vi "Begin.vi"(8 "error in (no error)":errorcluster, 10 "Config In":variant, 11 "TalonSRX in":refnum<class "TalonSRX.lvclass">) -> (0 "error out":errorcluster, 3 "TalonSRX out":refnum<class "TalonSRX.lvclass">)   [LabVIEW 2019, in "Drive.lvlib" / "TalonSRX.lvclass"]
uses:
  TalonSRX.lvclass
  C:/Users/Public/Documents/2020InfiniteRecharge/src robot/Classes/Drive/Tank Drive/Tank Drive.lvclass
  CTRE Drive.lvclass
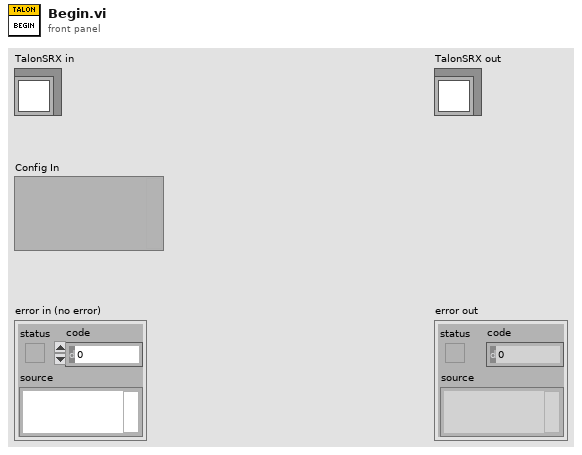
[diagram p1: front panel]
types:
  T1 = typedef "Drive.lvlib/Tank Drive.lvclass/Motor Controller IDs.ctl" = cluster{"Left Lead":u8, "Right Lead":u8, "Left Followers":u8[], "Right Followers":u8[]}
  T2 = typedef "Drive.lvlib/Tank Drive.lvclass/Motor Controller Names.ctl" = cluster{"Left Lead":string, "Right Lead":string, "Left Followers":string[], "Right Followers":string[]}
  T3 = typedef "CTRE_Phoenix_MotorControl_SlotStructure.ctl" = cluster{"P":dbl, "I":dbl, "D":dbl, "F":dbl, "integralZone":dbl, "allowableClosedLoopError":i32, "maxIntegralAccumulator":dbl, "closedLoopPeakOutput":dbl, "closedLoopPeriod":i32}
  T4 = typedef "DriveOld.lvlib/Drive.lvclass/Drive Sensor Data.ctl" = cluster{"Drive Right Invert":bool, "Drive Right Sensor Phase":bool, "Drive Left Invert":bool, "Drive Left Sensor Phase":bool}
  T5 = typedef "DriveOld.lvlib/Drive.lvclass/Motion Magic Constants.ctl" = cluster{"Low Gear Max Velocity":u32, "High Gear Max Velocity":u32, "Motion Magic Low Gear Max Velocity":u32, "Motion Magic Low Gear Max Acceleration":u32, "Motion Magic High Gear Max Velocity":u32, "Motion Magic High Gear Max Acceleration":u32}
  T6 = cluster{"Drive Velocity Low Gear":T3, "Drive Velocity High Gear":T3, "Drive Motion Magic Primary Low Gear":T3, "Drive Motion Magic Primary High Gear":T3, "Drive Motion Magic Secondary Low Gear":T3, "Drive Motion Magic Secondary High Gear":T3, "Drive Sensors":T4, "Motion Magic Constants":T5}
  T7 = typedef "WPI_MotorControlDeviceRef.ctl" = cluster{"DeviceStatus":errorcluster, "Type":T8, "PWM":cluster{"PWM Channel":T9, "DeadBand":T10}, "CAN":cluster{"Device Number":u8, "SetOutput VI Ref":variant, "GetOutput VI Ref":variant, "Enable VI Ref":variant, "Disable VI Ref":variant, "Data":variant}, "Invert":bool, "DIO PWM":cluster{"PWM \"Enable\" Channel":T9, "DIOChannel":T11, "PWM Rate":dbl}}
  T8 = typedef "WPI_MotorControlType.ctl" = enum16{"PWM", "CAN", "DIO PWM"}
  T9 = typedef "FPGA_DIOPWMChannel.ctl" = enum8{"PWM 0", "PWM 1", "PWM 2", "PWM 3", "PWM 4", "PWM 5", "PWM 6", "PWM 7", "PWM 8", "PWM 9", "PWM MXP 0", "PWM MXP 1", "PWM MXP 2", "PWM MXP 3", "PWM MXP 4", "PWM MXP 5", "PWM MXP 6", "PWM MXP 7", "PWM MXP 8", "PWM MXP 9", "Invalid"}
  T10 = typedef "WPI_PWMDeadband.ctl" = cluster{"Name":string, "maxPositivePwm":i32, "minPositivePwm":i32, "centerPwm":i32, "maxNegativePwm":i32, "minNegativePwm":i32, "angularRange":u16}
  T11 = typedef "FPGA_DIOChannel.ctl" = enum8{"DIO 0", "DIO 1", "DIO 2", "DIO 3", "DIO 4", "DIO 5", "DIO 6", "DIO 7", "DIO 8", "DIO 9", "DIO MXP 0", "DIO MXP 1", "DIO MXP 2", "DIO MXP 3", "DIO MXP 4", "DIO MXP 5", "DIO MXP 6", "DIO MXP 7", "DIO MXP 8", "DIO MXP 9", "DIO MXP 10", "DIO MXP 11", "DIO MXP 12", "DIO MXP 13", "DIO MXP 14", "DIO MXP 15", "SPI Port CS1", "SPI Port CS2", "SPI Port CS3", "SPI Port MISO", "SPI Port MOSI", "Invalid"}
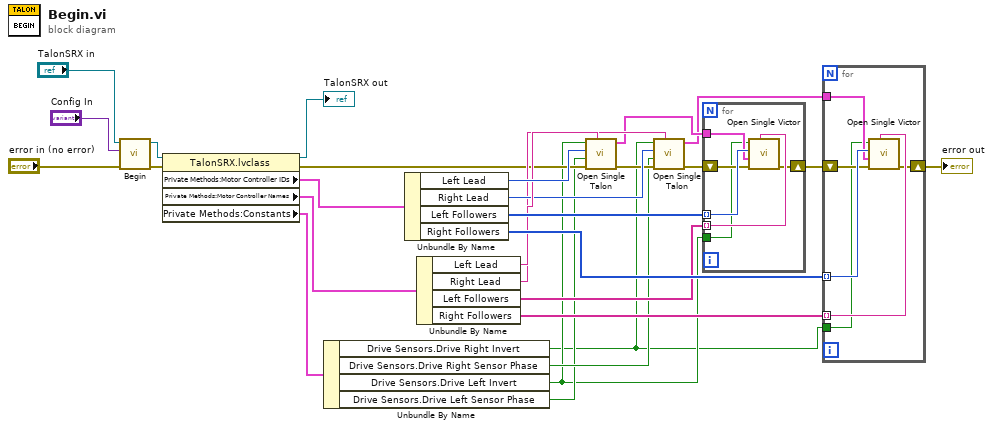
[diagram p0: block diagram]
diagram:
  n1 = call-parent "Begin.vi"("error in (no error)"="error in (no error)", "Config In"="Config In", "Tank Drive in"="TalonSRX in") -> ("error out"=w26:errorcluster, "Tank Drive out"=w25:refnum<class "TalonSRX.lvclass">)  [unwired: 7 in]
  n2 = property class="TalonSRX.lvclass"(reference=w25, error in=w26) -> (reference out=→"TalonSRX out":refnum<class "TalonSRX.lvclass">, error out=w9:errorcluster, "Private Methods:Motor Controller IDs"=w23:T1, "Private Methods:Motor Controller Names"=w22:T2, "Private Methods:Constants"=w5:T6)
  n3 = Unbundle By Name(w5) -> ("Drive Sensors.Drive Right Invert"=w1:bool, "Drive Sensors.Drive Right Sensor Phase"=w4:bool, "Drive Sensors.Drive Left Invert"=w2:bool, "Drive Sensors.Drive Left Sensor Phase"=w3:bool)
  n4 = Unbundle By Name(w23) -> ("Left Lead"=w17:u8, "Right Lead"=w15:u8, "Left Followers"=w21:u8[], "Right Followers"=w20:u8[])
  n5 = Unbundle By Name(w22) -> ("Left Lead"=w16:string, "Right Lead"=w14:string, "Left Followers"=w19:string[], "Right Followers"=w18:string[])
  n6 = call "Open Single Talon.vi"("refnum name"=w16, "error in (no error)"=w9, "sensor phase"=w3, "can id"=w17, "invert"=w2) -> ("error out"=w13:errorcluster, "PhoenixMotorControlDevRef"=w7:T7)  [unwired: 5 in]
  n7 = call "Open Single Talon.vi"("refnum name"=w14, "error in (no error)"=w13, "sensor phase"=w4, "can id"=w15, "invert"=w1) -> ("error out"=w12:errorcluster, "PhoenixMotorControlDevRef"=w6:T7)  [unwired: 5 in]
  n8 = for {
    tunnel: w21 -> [w34] mode=indexing
    tunnel: w19 -> [w33] mode=indexing
    shift-right: [w31] -> w11
    shift-left: w12 -> [w32]
    tunnel: w7 -> [w30]
    tunnel: w2 -> [w29]
    n9 = call "Open Single Victor.vi"("refnum name"=w33, "error in (no error)"=w32, "Master Controller to Follow"=w30, "Device Number"=w34, "Invert?"=w29) -> ("error out"=w31:errorcluster)  [unwired: 6 in]
  }
  n10 = for {
    tunnel: w20 -> [w40] mode=indexing
    tunnel: w18 -> [w39] mode=indexing
    shift-right: [w37] -> w8
    shift-left: w11 -> [w38]
    tunnel: w6 -> [w36]
    tunnel: w1 -> [w35]
    n11 = call "Open Single Victor.vi"("refnum name"=w39, "error in (no error)"=w38, "Master Controller to Follow"=w36, "Device Number"=w40, "Invert?"=w35) -> ("error out"=w37:errorcluster)  [unwired: 6 in]
  }
  "error out" <- w8
